vi "Get Speed Info.vi"(10 "Velocity in":T1, 11 "Movable in":refnum<class "Movable.lvclass">) -> (2 "Max speed?":bool, 4 "ratio out":dbl)   [LabVIEW 2024, in "Movable.lvclass"]
doc: "MIT Licence\nCopyright (c) 2024 David Grollier"
uses:
  Movable.lvclass
  Type Def/Velocity.ctl
  Movable.lvclass/Movable.ctl
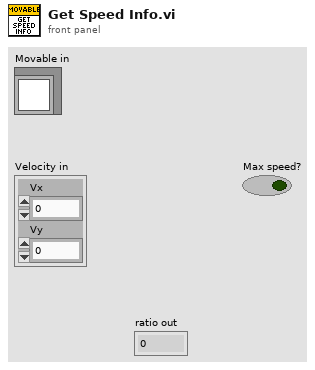
[diagram p1: front panel]
types:
  T1 = typedef "Velocity.ctl" = cluster{"Vx":dbl, "Vy":dbl}
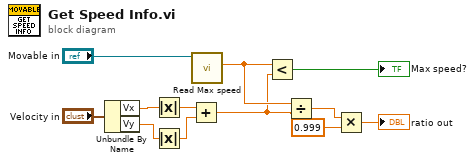
[diagram p0: block diagram]
diagram:
  n1 = Unbundle By Name("Velocity in") -> ("Vx"=w8:dbl, "Vy"=w7:dbl)
  n2 = Absolute Value(x=w8) -> (abs(x)=w11:dbl)
  n3 = Absolute Value(x=w7) -> (abs(x)=w10:dbl)
  n4 = Add(x=w11, y=w10) -> (x+y=w4:dbl)
  n5 = call "Read Max speed.vi"("Movable in"="Movable in") -> ("Max speed"=w5:dbl)  [unwired: 10 in]
  n6 = Less?(x=w5, y=w4) -> (x < y?=→"Max speed?":bool)
  n7 = Divide(x=w5, y=w4) -> (x/y=w3:dbl)
  n8 = Multiply(x=w3, y=0.999) -> (x*y=→"ratio out":dbl)
